vi "HXG2_VerifyPath.vi"(8 "error in (no error)":errorcluster, 11 "Path In":path) -> (0 "error out":errorcluster, 3 "Path Out":path)   [LabVIEW 2012]
doc: "Verify if path/folder exists, if not, create it."
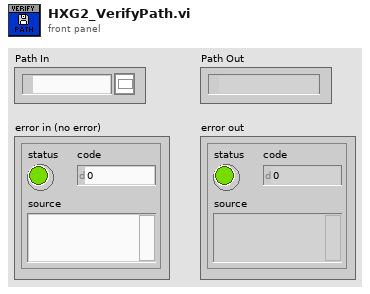
[diagram p1: front panel]
types:
  T1 = enum16{"open", "replace", "create", "open or create", "replace or create", "replace or create with confirmation"}
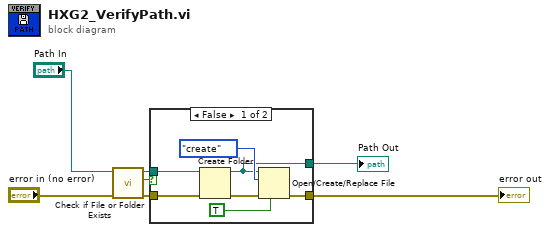
[diagram p0: block diagram]
diagram:
  n1 = call <vilib>:"Check if File or Folder Exists.vi"("error in (no error)"="error in (no error)", "path"="Path In") -> ("error out"=w3:errorcluster, "file or folder exists?"=w5:bool, "dup path"=w6:path)  [unwired: 7 in]
  n2 = case shown="False" w5 {
    tunnel: w3 -> [w14 w15]
    tunnel: w6 -> [w13 w16]
    tunnel: [w11 w15] -> w1
    tunnel: [w8 w16] -> w7
    frame False {
      n3 = Create Folder(path (use dialog)=w13, error in=w14) -> (created path=w8:path, error out=w12:errorcluster)  [unwired: 1 in, 1 out]
      n4 = Open/Create/Replace File(file path (use dialog)=w8, error in=w12, operation (0:open)=T1."create", disable buffering (F)=TRUE) -> (error out=w11:errorcluster)  [unwired: 2 in, 2 out]
    }
    frame True {
    }
  }
  "Path Out" <- w7
  "error out" <- w1
